vi "Read String Range.vi"(0 "Report Ref In":T1, 1 "Row Count":i32=1, 2 "Start Row Index":i32, 3 "Start Column Index":i32, 4 "Column Count":i32=1, 5 "error in (no error)":errorcluster) -> (6 "Report Ref Out":T1, 7 "Output Range":string[][](array[string]), 8 "error out":errorcluster)   [LabVIEW 2013, in "XCel Report Engine.lvlib"]
doc: "Reads a rectangular range of cells from the active worksheet and returns the values as a two-dimensional string array.\n\nThe range is specified by zero-based starting row and column coordinates together with the number of rows and columns. Coordinate (0, 0) corresponds to cell A1.\n\nEmpty or missing cells are returned as empty strings. Boolean and numeric values are converted using the same rules as Read Cell String.vi.\n\nIf any cell in the requested range contains a formula, the entire operation returns an error. XCelReportEngine does not evaluate formulas or return cached formula results.\n\nRow Count and Column Count must both be greater than zero, and the requested range must remain within the Excel worksheet limits."
uses:
  XCel Report Engine.lvlib
  C:/Users/m.santucci/Documents/ChatGPT/LV_REPORT_ENGINE/LV/DotNet/XCelReportEngine.dll
  LV/DotNet/XCelReportEngine.dll
  Controls/Report Ref.ctl
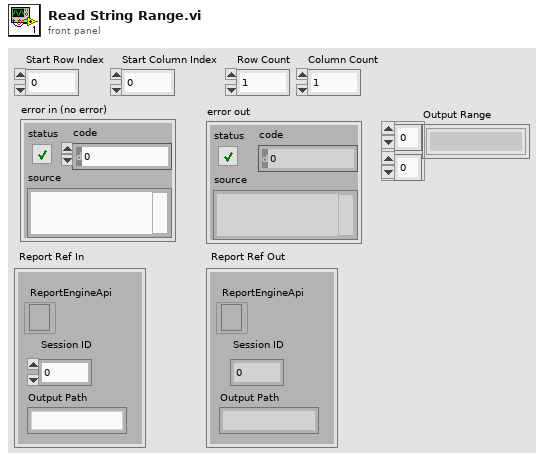
[diagram p1: front panel]
types:
  T1 = typedef "XCel Report Engine.lvlib/Report Ref.ctl" = cluster{"Session ID":i32, "Output Path":string, "ReportEngineApi":refnum<k24>}
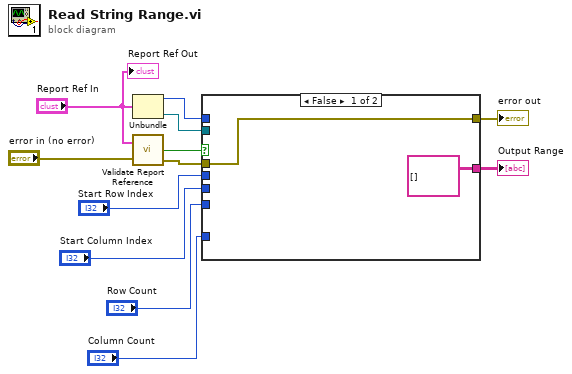
[diagram p0: block diagram]
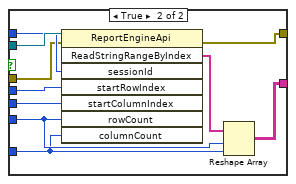
[diagram p2: hidden frame]
diagram:
  n1 = Unbundle("Report Ref In") -> ("Session ID"=w10:i32, "ReportEngineApi"=w12:refnum<k24>)  [unwired: 1 out]
  n2 = call "Validate Report Reference.vi"("Report Ref In"="Report Ref In", "error in (no error)"="error in (no error)") -> ("Valid"=w1:bool, "error out"=w2:errorcluster)  [unwired: 1 out]
  n3 = case shown="False" w1 {
    tunnel: w12 -> [_ w24]
    tunnel: [w14 w23] -> w11
    tunnel: w10 -> [_ w22]
    tunnel: "Start Row Index" -> [_ w21]
    tunnel: "Start Column Index" -> [_ w20]
    tunnel: "Row Count" -> [_ w18]
    tunnel: "Column Count" -> [_ w17]
    tunnel: [string[][] [] ("ReadStringRangeByIndex") w16] -> w5
    tunnel: w2 -> [w14 w15]
    frame False {
    }
    frame True {
      n4 = invoke class="ReportEngineApi" method="ReadStringRangeByIndex"(reference=w24, error in=w15, "sessionId"=w22, "startRowIndex"=w21, "startColumnIndex"=w20, "rowCount"=w18, "columnCount"=w17) -> (error out=w23:errorcluster, "ReadStringRangeByIndex"=w19:string[])  [unwired: 1 in, 6 out]
      n5 = Reshape Array(w19, w18, w17) -> (w16:string[][])
    }
  }
  "error out" <- w11
  "Output Range" <- w5
  "Report Ref Out" <- "Report Ref In"
